vi "Define 2D Helmholtz PDE Domain (Polygon).vi"(0 "PDE in":refnum<class "NI_PDE.lvclass">, 1 "grid factor":dbl=0.005, 5 "Boundary Points":cluster{"X":dbl, "Y":dbl}[](array[cluster]), 7 "Grid Points":cluster{"X":dbl, "Y":dbl}[](array[cluster]), 11 "error in (no error)":errorcluster) -> (4 "PDE out":refnum<class "NI_PDE.lvclass">, 15 "error out":errorcluster)   [LabVIEW 2020, in "NI_PDE.lvlib"]
doc: "Defines the domain where you solve the partial differential equation. You must manually select the polymorphic instance to use."
uses:
  <vilib>/gmath/NI_PDE.lvlib
  <vilib>/gmath/pde.llb/PDEClass/NI_PDE.lvclass
  <vilib>/gmath/pde.llb/PDEClass/PDE_Helmholtz_2D/NI_PDE_Helmholtz_2D.lvclass
  e:/builds/penguin/labview/branches/2020/dev/dist/vi.lib/gmath/pde.llb/PDEClass/NI_PDE.lvclass
  <vilib>/gmath/pde.llb/DomainClass/Domain_Steady_2D_Polygon/NI_Domain_Steady_2D_Polygon.lvclass
  e:/builds/penguin/labview/branches/2020/dev/dist/vi.lib/gmath/pde.llb/DomainClass/NI_Domain.lvclass
  <vilib>/gmath/pde.llb/DomainClass/Domain_Steady_2D_Polygon/Domain Data.ctl
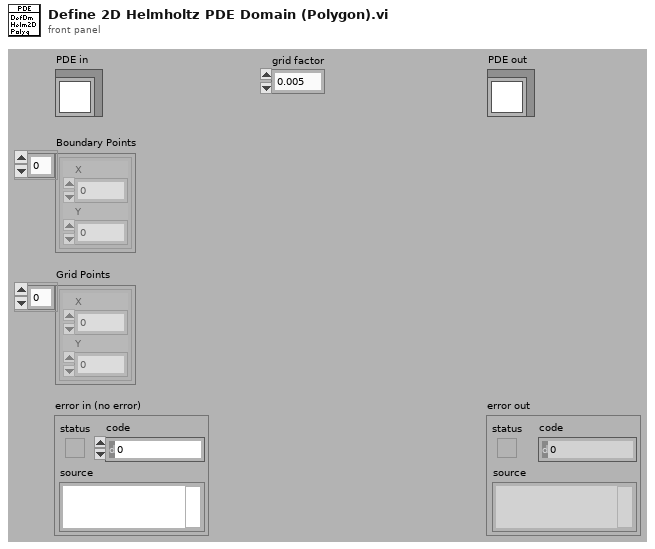
[diagram p1: front panel]
types:
  T1 = typedef "NI_PDE.lvlib/NI_Domain_Steady_2D_Polygon.lvclass/Domain Data.ctl" = cluster{"X":dbl[], "Y":dbl[], "Xi":dbl[], "Yi":dbl[], "grid factor":dbl, "Triangulation":i32[][]}
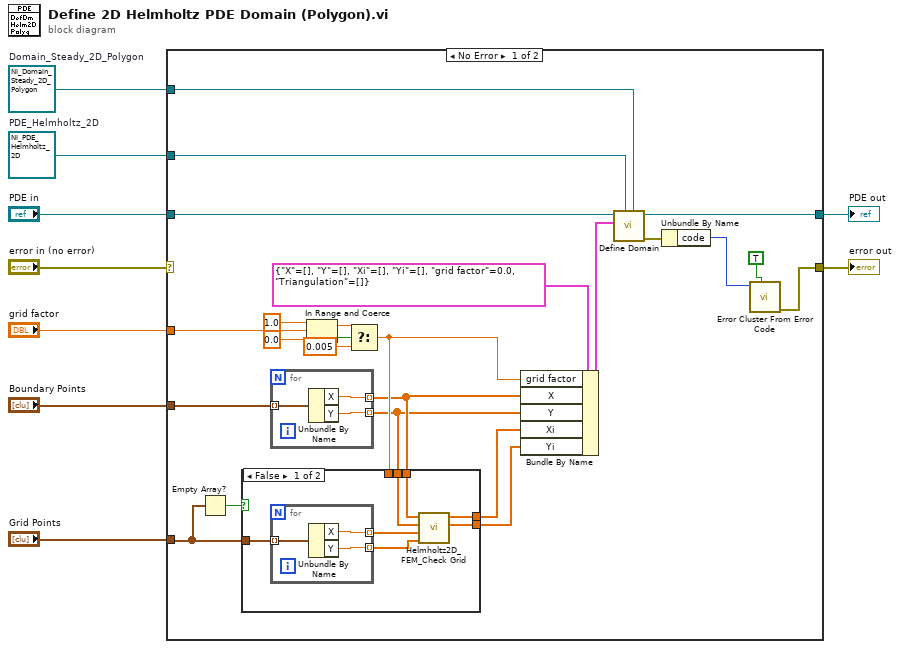
[diagram p0: block diagram]
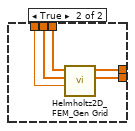
[diagram p2: hidden frame]
diagram:
  w1 = refnum<class "NI_Domain_Steady_2D_Polygon.lvclass"> refnum  # Domain_Steady_2D_Polygon
  w2 = refnum<class "NI_PDE_Helmholtz_2D.lvclass"> refnum  # PDE_Helmholtz_2D
  n1 = case shown="No Error" "error in (no error)" {
    selector: "error in (no error)" -> [_ w53]
    tunnel: "PDE in" -> [w10 w52]
    tunnel: [w13 w52] -> w8
    tunnel: "grid factor" -> [w25 _]
    tunnel: "Boundary Points" -> [w22 _]
    tunnel: "Grid Points" -> [w23 _]
    tunnel: [w31 w53] -> w4
    tunnel: w2 -> [w15 _]
    tunnel: w1 -> [w14 _]
    frame No Error {
      n2 = Empty Array?(array=w23) -> (empty?=w24:bool)
      n3 = for {
        tunnel: w22 -> [w36] mode=indexing
        tunnel: [w35] -> w19 mode=indexing
        tunnel: [w34] -> w18 mode=indexing
        n4 = Unbundle By Name(w36) -> ("X"=w35:dbl, "Y"=w34:dbl)
      }
      n5 = In Range and Coerce(upper limit=1.0, x=w25, lower limit=0.0) -> (coerced(x)=w27:dbl, In Range?=w26:bool)
      n6 = Select(t=w27, s=w26, f=0.005) -> (s? t:f=w20:dbl)
      n7 = case shown="False" w24 {
        tunnel: [w40 w51] -> w17
        tunnel: [w39 w50] -> w16
        tunnel: w20 -> [_ w49]
        tunnel: w19 -> [w42 w48]
        tunnel: w18 -> [w41 w47]
        tunnel: w23 -> [w43 _]
        frame False {
          n8 = for {
            tunnel: w43 -> [w46] mode=indexing
            tunnel: [w45] -> w38 mode=indexing
            tunnel: [w44] -> w37 mode=indexing
            n9 = Unbundle By Name(w46) -> ("X"=w45:dbl, "Y"=w44:dbl)
          }
          n10 = call <vilib>:"Helmholtz2D_FEM_Check Grid.vi"("Yi In"=w37, "Xi In"=w38, "Y"=w41, "X"=w42) -> ("Yi Out"=w39:dbl[], "Xi Out"=w40:dbl[])  [unwired: 6 out]
        }
        frame True {
          n11 = call <vilib>:"Helmholtz2D_FEM_Gen Grid.vi"("grid factor"=w49, "Y"=w47, "X"=w48) -> ("Yi"=w50:dbl[], "Xi"=w51:dbl[])  [unwired: 7 out]
        }
      }
      n12 = Bundle By Name(cluster=T1 {"X"=[], "Y"=[], "Xi"=[], "Yi"=[], "grid factor"=0.0, "Triangulation"=[]} ("domain data"), "grid factor"=w20, "X"=w19, "Y"=w18, "Xi"=w17, "Yi"=w16) -> (w11:T1)
      n13 = call <vilib>:"Define Domain.vi"("target Domain"=w14, "target PDE"=w15, "domain"=w11, "PDE in"=w10) -> ("error out"=w12:errorcluster, "PDE out"=w13:refnum<class "NI_PDE.lvclass">)  [unwired: 1 in, 5 out]
      n14 = Unbundle By Name(w12) -> ("code"=w33:i32)
      n15 = call <vilib>:"Error Cluster From Error Code.vi"("show call chain? (False)"=TRUE, "error code (0)"=w33) -> ("error out"=w31:errorcluster)  [unwired: 1 in, 6 out]
    }
    frame Error {
    }
  }
  "PDE out" <- w8
  "error out" <- w4
